vi "Next.vi"(8 "error in (no error)":errorcluster, 11 "LUnit Test Suite In":refnum<class "LUnit Test Suite.lvclass">) -> (0 "error out":errorcluster, 2 "Next Runnable":string, 3 "LUnit Test Suite Out":refnum<class "LUnit Test Suite.lvclass">)   [LabVIEW 2020, in "LUnit Test Suite.lvclass"]
doc: "Get next active test in suite. This works recursively for nested suites."
uses:
  LUnit Test Suite.lvclass
  LUnit Test Suite.lvclass/LUnit Test Suite.ctl
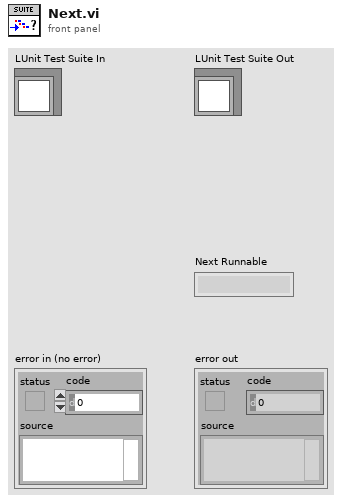
[diagram p1: front panel]
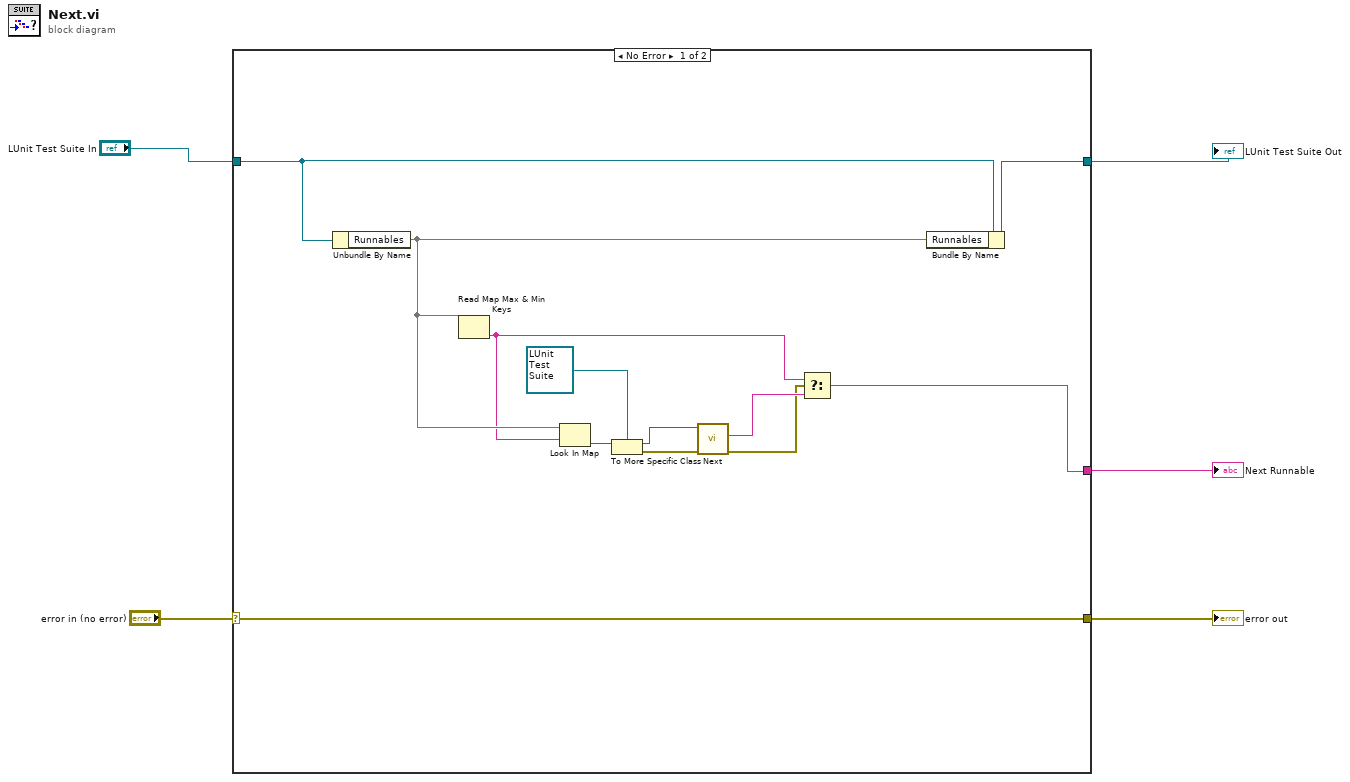
[diagram p0: block diagram]
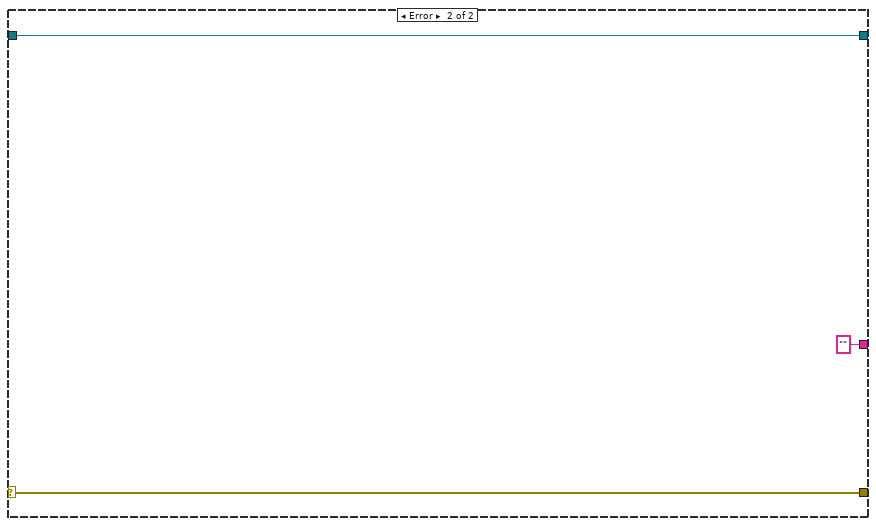
[diagram p2: hidden frame]
diagram:
  n1 = case shown="No Error" "error in (no error)" {
    selector: "error in (no error)" -> [w6 w20]
    tunnel: "LUnit Test Suite In" -> [w17 w19]
    tunnel: [w16 w19] -> w4
    tunnel: [w15 "" ("Next Runnable")] -> w3
    tunnel: [w6 w20] -> w1
    frame No Error {
      n2 = Unbundle By Name(w17) -> ("Runnables"=w14:map{string, refnum<class "Runnable.lvclass">})
      n3 = Read Map Max & Min Keys(11:w14) -> (1:w12:string)  [unwired: 1 out]
      n4 = Look In Map(map=w14, key=w12) -> (value=w13:refnum<class "Runnable.lvclass">)  [unwired: 1 in, 1 out]
      n5 = To More Specific Class(target class=refnum<class "LUnit Test Suite.lvclass"> refnum ("LUnit Test Suite Out"), reference=w13) -> (specific class reference=w11:refnum<class "LUnit Test Suite.lvclass">, error out=w9:errorcluster)  [unwired: 1 in]
      n6 = call "Next.vi"("error in (no error)"=w9, "LUnit Test Suite In"=w11) -> ("error out"=w7:errorcluster, "Next Runnable"=w8:string)  [unwired: 7 in, 1 out]
      n7 = Select(t=w12, s=w7, f=w8) -> (s? t:f=w15:string)
      n8 = Bundle By Name(cluster=w17, "Runnables"=w14) -> (w16:refnum<class "LUnit Test Suite.lvclass">)
    }
    frame Error {
    }
  }
  "error out" <- w1
  "LUnit Test Suite Out" <- w4
  "Next Runnable" <- w3
